vi "Get Dashboard Data.vi"   [LabVIEW 2012]
uses:
  BotStatus.vi
types:
  T1 = cluster{"Target Position X":dbl, "Target Position Y":dbl, "Target Found":bool}
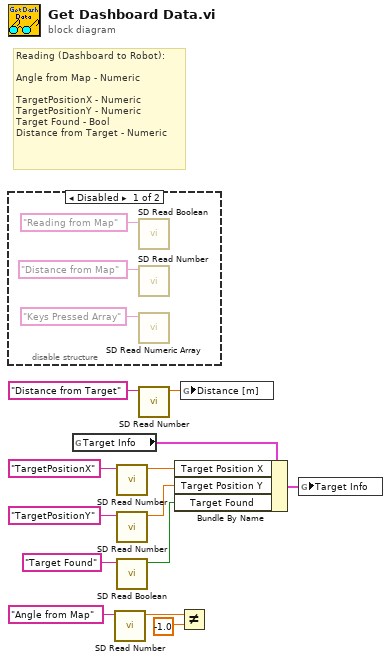
[diagram p0: block diagram]
diagram:
  # "Reading (Dashboard to Robot):\n\nAngle from Map - Numeric\n\nTargetPositionX - Numeric\nTargetPositionY - Numeric\nTarget Found - Bool\nDistance from Target - Numeric"
  n1 = disable-structure shown="Disabled" {
    frame Disabled {
      n2 = call <vilib>:"SD Read Boolean.vi"("Name"="Reading from Map") -> ()  [unwired: 8 in, 3 out]
      n3 = call <vilib>:"SD Read Number.vi"("Name"="Distance from Map") -> ()  [unwired: 8 in, 3 out]
      n4 = call <vilib>:"SD Read Numeric Array.vi"("Name"="Keys Pressed Array") -> ()  [unwired: 8 in, 3 out]
    }
    frame Enabled {
    }
  }
  n5 = global read "BotStatus.vi" "Target Info"() -> (w9:T1)
  n6 = call <vilib>:"SD Read Number.vi"("Name"="Angle from Map") -> ("Numeric"=w2:dbl)  [unwired: 8 in, 2 out]
  n7 = call <vilib>:"SD Read Number.vi"("Name"="TargetPositionX") -> ("Numeric"=w8:dbl)  [unwired: 8 in, 2 out]
  n8 = call <vilib>:"SD Read Number.vi"("Name"="TargetPositionY") -> ("Numeric"=w7:dbl)  [unwired: 8 in, 2 out]
  n9 = call <vilib>:"SD Read Boolean.vi"("Name"="Target Found") -> ("Boolean"=w6:bool)  [unwired: 8 in, 2 out]
  n10 = call <vilib>:"SD Read Number.vi"("Name"="Distance from Target") -> ("Numeric"=w4:dbl)  [unwired: 8 in, 2 out]
  n11 = Bundle By Name(cluster=w9, "Target Position X"=w8, "Target Position Y"=w7, "Target Found"=w6) -> (w5:T1)
  n12 = Not Equal?(x=w2, y=-1.0) -> ()  [unwired: 1 out]
  n13 = global write "BotStatus.vi" "Distance [m]"(w4) -> ()
  n14 = global write "BotStatus.vi" "Target Info"(w5) -> ()
